vi "SetGlobalVariables.vi"(8 "error in (no error)":errorcluster, 11 "xckdelay":u32) -> (0 "error out":errorcluster)   [LabVIEW 2015, in "ESLSCDLL.lvlib"]
uses:
  ESLSCDLL.lvlib
  Globals.vi
  ESLSCDLL.dll
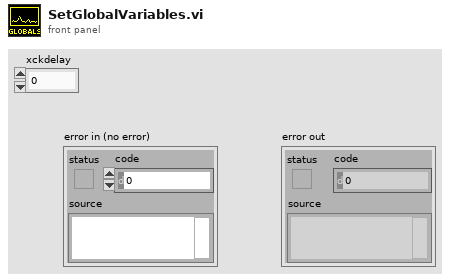
[diagram p1: front panel]
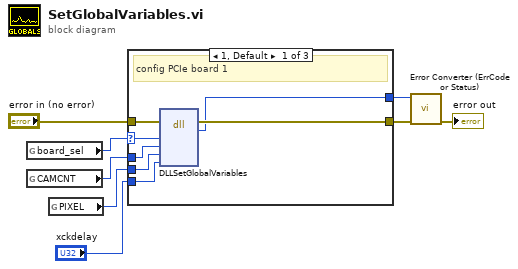
[diagram p0: block diagram]
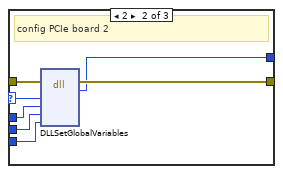
[diagram p2: hidden frame]
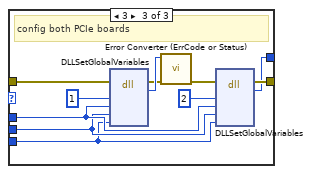
[diagram p3: hidden frame]
diagram:
  n1 = global read "Globals.vi" "board_sel"() -> (w4:u32)
  n2 = global read "Globals.vi" "CAMCNT"() -> (w3:u32)
  n3 = global read "Globals.vi" "PIXEL"() -> (w2:u32)
  n4 = case shown="1, Default" w4 {
    selector: w4 -> [w15 w20 _]
    tunnel: "error in (no error)" -> [w14 w21 w28]
    tunnel: [w13 w22 w32] -> w6
    tunnel: [w12 w19 w31] -> w5
    tunnel: w3 -> [w11 w18 w25]
    tunnel: w2 -> [w10 w17 w24]
    tunnel: "xckdelay" -> [w9 w16 w23]
    frame 1, Default {
      # "config PCIe board 1"
      n5 = dll-call lib="C:/ENTW/PCIE/LV64/board.vis/ESLSCDLL.dll" fn="DLLSetGlobalVariables" ("lwlscdll.dll:DLLSetupVCLK")(error in=w14, "drvno"=w15, "camcnt"=w11, "pixel"=w10, "xckdelay"=w9) -> (error out=w13:errorcluster, "es_status_codes"=w12:i32)  [unwired: 6 in, 1 out]
    }
    frame 2 {
      # "config PCIe board 2"
      n6 = dll-call lib="C:/ENTW/PCIE/LV64/board.vis/ESLSCDLL.dll" fn="DLLSetGlobalVariables" ("lwlscdll.dll:DLLSetupVCLK")(error in=w21, "drvno"=w20, "camcnt"=w18, "pixel"=w17, "xckdelay"=w16) -> (error out=w22:errorcluster, "es_status_codes"=w19:i32)  [unwired: 6 in, 1 out]
    }
    frame 3 {
      # "config both PCIe boards"
      n7 = dll-call lib="C:/ENTW/PCIE/LV64/board.vis/ESLSCDLL.dll" fn="DLLSetGlobalVariables" ("lwlscdll.dll:DLLSetupVCLK")(error in=w28, "drvno"=u32 1, "camcnt"=w25, "pixel"=w24, "xckdelay"=w23) -> (error out=w29:errorcluster, "es_status_codes"=w30:i32)  [unwired: 6 in, 1 out]
      n8 = call "Error Converter (ErrCode or Status).vi"("error in (no error)"=w29, "error code"=w30) -> ("error out"=w33:errorcluster)  [unwired: 9 in]
      n9 = dll-call lib="C:/ENTW/PCIE/LV64/board.vis/ESLSCDLL.dll" fn="DLLSetGlobalVariables" ("lwlscdll.dll:DLLSetupVCLK")(error in=w33, "drvno"=u32 2, "camcnt"=w25, "pixel"=w24, "xckdelay"=w23) -> (error out=w32:errorcluster, "es_status_codes"=w31:i32)  [unwired: 6 in, 1 out]
    }
  }
  n10 = call "Error Converter (ErrCode or Status).vi"("error in (no error)"=w6, "error code"=w5) -> ("error out"=→"error out":errorcluster)  [unwired: 9 in]
